vi "Locate speed data folder.vi"(8 "error in (no error)":errorcluster, 11 "Value":path) -> (0 "error out":errorcluster, 3 "Speed data folder's path":path)   [LabVIEW 2020]
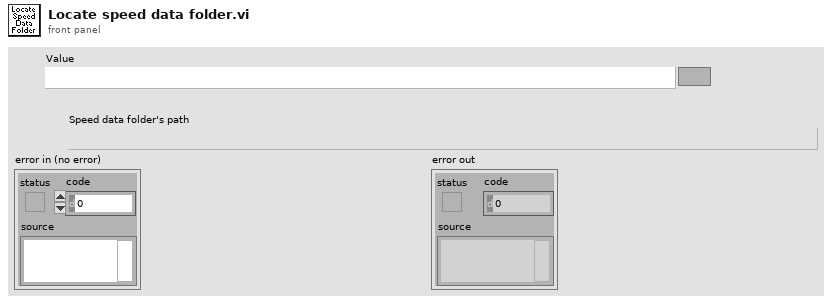
[diagram p1: front panel]
types:
  T1 = typedef "Fixed strings.ctl" = cluster{"ROI file name":string, "Normalised ROI file name":string, "Zplane Pockels values file name":string, "Functional data folder name":string, "Experiment Header file name":string, "Z-stack images folder name":string, "Groups setup rel. path":string, "Groups text file rel. path":string, "TDMS files folder name (F.img)":string, "TDMS files folder name (V.acq)":string, "TDMS files folder name (Pl.acq)":string, "Cycle rel times sequence file":string, "Dynamically called VIs folder name":string, "Time Series folder base name":string}
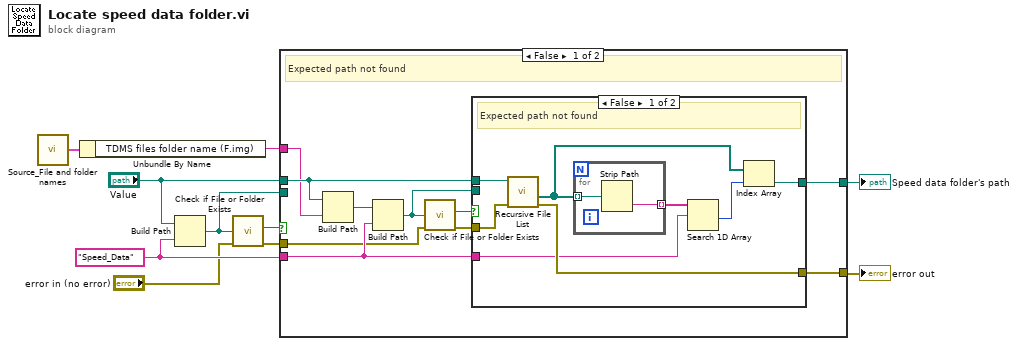
[diagram p0: block diagram]
diagram:
  w7 = "Speed_Data" ("name or relative path")
  n1 = call "Source_File and folder names.vi"() -> ("Fixed strings"=w2:T1)  [unwired: 1 in]
  n2 = Unbundle By Name(w2) -> ("TDMS files folder name (F.img)"=w1:string)
  n3 = Build Path(base path="Value", name or relative path=w7) -> (appended path=w4:path)
  n4 = call <vilib>:"Check if File or Folder Exists.vi"("error in (no error)"="error in (no error)", "path"=w4) -> ("error out"=w3:errorcluster, "file or folder exists?"=w6:bool)  [unwired: 7 in, 1 out]
  n5 = case shown="False" w6 {
    tunnel: [w20 w34] -> w10
    tunnel: "Value" -> [w18 _]
    tunnel: [w19 w33] -> w9
    tunnel: w3 -> [w12 w33]
    tunnel: w7 -> [w15 _]
    tunnel: w4 -> [_ w34]
    tunnel: w1 -> [w17 _]
    frame False {
      # "Expected path not found"
      n6 = Build Path(base path=w18, name or relative path=w17) -> (appended path=w16:path)
      n7 = Build Path(base path=w16, name or relative path=w15) -> (appended path=w13:path)
      n8 = call <vilib>:"Check if File or Folder Exists.vi"("error in (no error)"=w12, "path"=w13) -> ("error out"=w11:errorcluster, "file or folder exists?"=w14:bool)  [unwired: 7 in, 1 out]
      n9 = case shown="False" w14 {
        tunnel: [w28 w32] -> w20
        tunnel: w18 -> [w25 _]
        tunnel: [w24 w31] -> w19
        tunnel: w11 -> [w23 w31]
        tunnel: w15 -> [w21 _]
        tunnel: w13 -> [_ w32]
        frame False {
          # "Expected path not found"
          n10 = call <vilib>:"Recursive File List.vi"("error in (no error)"=w23, "Folder Path"=w25) -> ("error out"=w24:errorcluster, "All Folders"=w22:path[])  [unwired: 5 in, 3 out]
          n11 = for {
            tunnel: w22 -> [w30] mode=indexing
            tunnel: [w29] -> w26 mode=indexing
            n12 = Strip Path(path=w30) -> (name=w29:string)  [unwired: 1 out]
          }
          n13 = Search 1D Array(1D array=w26, element=w21) -> (index of element=w27:i32)  [unwired: 1 in]
          n14 = Index Array(array=w22, index=w27) -> (element=w28:path)
        }
        frame True {
          # "Expected path found"
        }
      }
    }
    frame True {
      # "Expected path found"
    }
  }
  "Speed data folder's path" <- w10
  "error out" <- w9
